vi "DiscArchiver.new event data.vi"(0 "i ref":refnum<vi>, 1 "eventData":string, 2 "descriptor":string, 3 "ms timeout (10000)":i32=10000, 5 "error in (no error)":errorcluster) -> (14 "i ref out":refnum<vi>, 17 "timed out":bool, 19 "error out":errorcluster)   [LabVIEW 2014, in "DiscArchiver.lvlib"]
doc: "The method is executed, when new event data is received. The data will be written to file."
uses:
  DiscArchiver.lvlib
  CS_Core/CSSystem/CoreDefs/CoreDefs.rawDataType.ctl
  CS_Core/CSSystem/CoreDefs/CoreDefs.error_type.ctl
  CS_Core/CSSystem/CoreDefs/CoreDefs.error_severity.ctl
  DataLib/DataLib.lvlib
  CS_Core/CSSystem/CoreLib/CoreLib.lvlib
  CSlibraries-extern/DimLVEvent/LVDimInterface/LVDimInterface.lvlib
  CSlibraries/UtilityLib/UtilityLib.lvlib
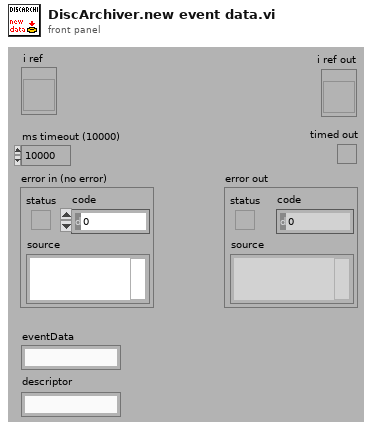
[diagram p1: front panel]
types:
  T1 = typedef "CoreDefs.rawDataType.ctl" = i8[]
  T2 = typedef "CoreDefs.error_severity.ctl" = enum16{"undefined", "information", "warning", "error", "fatal"}
  T3 = typedef "CoreDefs.error_type.ctl" = enum16{"no error", "can't load process", "can't unload process", "process does not exist", "can't install process", "can't remove process", "unknown function", "time out", "can't execute function", "duplicate queue name", "super not found", "caller queue invalid", "can't ping process", "unknown error", "VISA Error", "VISA timeout", "GPIB timeout", "GPIB error", "communication error", "data type mismatch", "can't read data from OPC server", "can't write data to OPC server", "OET error", "function not implemented", "process already exists", "invalid Shared Variable name", "error writing Shared Variable", "error reading Shared Variable", "invalid client name", "corrupt database", "unknown class", "call not authorized", "parameter out of range", "OET timeout: can't get data to modify", "invalid queue name", "requested operation incompatible with current state", "event undefined", "event disabled", "state undefined", "caller is not a friend", "EventBuilder: bad eventID", "EventBuilder: no DAQ devices", "a thread must not stop itself", "UNUSED ELEMENT4", "DiscArchiver: eventData incomplete", "DiscArchiver: eventData does not belong to run", "DiscArchiver: can't open file", "DiscArchiver: can't write to file", "DiscArchiver: available disc space low", "can't acquire semaphore", "error reading data from database", "notifier object is not existing", "can't register process", "can't unregister process", "illegal event type", "object disabled", "object already exists", "can't change state", "Instrument not found", "no connection to remote node", "invalid reference", "N/A", "UNUSED ELEMENT 1", "element not found", "illegal TCP/IP connection detected", "object does not exist", "invalid access ID", "unknown CS system", "invalid privilige", "unsupported data type", "unsupported server type", "IO server already exists", "Shared Variable already exists"}
  T4 = typedef "DiscArchiver.lvlib/DiscArchiver.i attribute.ctl" = cluster{"file prefix":string, "actual file":string, "nOfEvents":i32, "file":refnum<file>, "eventBuilder":string, "disc size alarm":bool, "dataDescription":string, "dataDescriptionURL":string, "eventDataURL":string, "headerID":dbl, "completeData":bool, "nOfEventsID":i32, "dataFileID":i32}
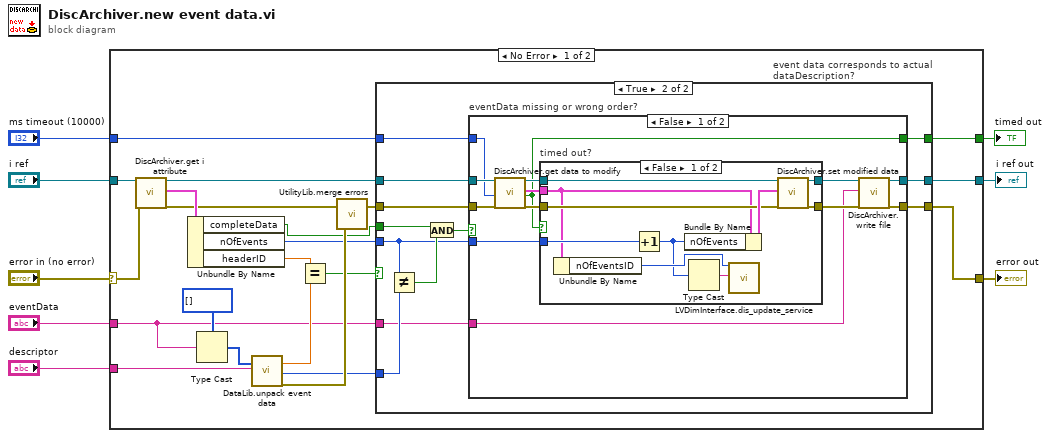
[diagram p0: block diagram]
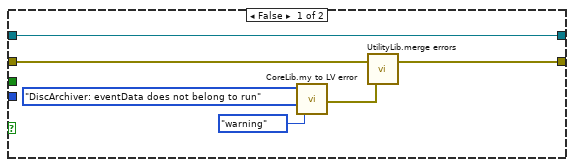
[diagram p2: hidden frame]
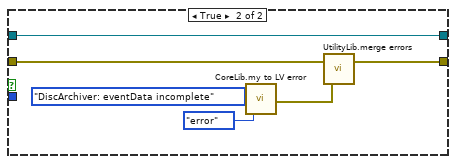
[diagram p4: hidden frame]
diagram:
  n1 = case shown="No Error" "error in (no error)" {
    selector: "error in (no error)" -> [w26 w79]
    tunnel: [w23 w79] -> w8
    tunnel: "eventData" -> [w9 _]
    tunnel: [w22 w80] -> w6
    tunnel: "i ref" -> [w27 w80]
    tunnel: "ms timeout (10000)" -> [w24 _]
    tunnel: "descriptor" -> [w17 _]
    tunnel: [w21 _] -> w2
    frame No Error {
      n2 = call "DiscArchiver.get i attribute.vi"("i ref in"=w27, "error in (no error)"=w26) -> ("i ref out"=w25:refnum<vi>, "i attribute"=w28:T4, "error out"=w15:errorcluster)  [unwired: 15 in]
      n3 = Unbundle By Name(w28) -> ("completeData"=w10:bool, "nOfEvents"=w12:i32, "headerID"=w29:dbl)
      n4 = Type Cast(type=T1 [] ("Array"), x=w9) -> (*(type *) &x=w20:T1)
      n5 = call "DataLib.unpack event data.vi"("serviceData"=w20, "descriptor"=w17) -> ("headerID"=w18:dbl, "eventID"=w11:i32, "error out"=w14:errorcluster)  [unwired: 13 in, 2 out]
      n6 = Equal?(x=w29, y=w18) -> (x = y?=w13:bool)
      n7 = call "UtilityLib.merge errors.vi"("error2 (no error)"=w14, "error1 (no error)"=w15) -> ("error out"=w16:errorcluster)
      n8 = case "event data corresponds to actual dataDescription?" shown="True" w13 {
        tunnel: w25 -> [w35 w47]
        tunnel: w16 -> [w32 w46]
        tunnel: w24 -> [_ w45]
        tunnel: [w33 w44] -> w23
        tunnel: [w35 w43] -> w22
        tunnel: [_ w42] -> w21
        tunnel: w12 -> [_ w37]
        tunnel: w11 -> [_ w41]
        tunnel: w10 -> [_ w40]
        tunnel: w9 -> [_ w36]
        frame False {
          n9 = call "CoreLib.my to LV error.vi"("ErrorTypes"=CoreDefs.error_type."DiscArchiver: eventData does not belong to run", "severityLevel"=CoreDefs.error_severity."warning") -> ("myErrorCluster"=w31:errorcluster)  [unwired: 16 in, 1 out]
          n10 = call "UtilityLib.merge errors.vi"("error2 (no error)"=w31, "error1 (no error)"=w32) -> ("error out"=w33:errorcluster)
        }
        frame True {
          n11 = Not Equal?(x=w37, y=w41) -> (x != y?=w39:bool)
          n12 = And(x=w40, y=w39) -> (x .and. y?=w38:bool)
          n13 = case "eventData missing or wrong order?" shown="False" w38 {
            tunnel: w47 -> [w60 w78]
            tunnel: w46 -> [w59 w76]
            tunnel: w45 -> [w53 _]
            tunnel: [w52 w77] -> w44
            tunnel: [w51 w78] -> w43
            tunnel: [w49 _] -> w42
            tunnel: w37 -> [w50 _]
            tunnel: w36 -> [w48 _]
            frame False {
              n14 = call "DiscArchiver.get data to modify.vi"("i ref in"=w60, "ms timeout (10000)"=w53, "error in (no error)"=w59) -> ("i ref out"=w58:refnum<vi>, "i attribute"=w57:T4, "timed out"=w49:bool, "error out"=w56:errorcluster)  [unwired: 13 in]
              n15 = case "timed out?" shown="False" w49 {
                tunnel: w58 -> [w70 w71]
                tunnel: w57 -> [w64 _]
                tunnel: w56 -> [w68 w72]
                tunnel: [w65 w72] -> w54
                tunnel: [w67 w71] -> w55
                tunnel: w50 -> [w66 _]
                frame False {
                  n16 = Unbundle By Name(w64) -> ("nOfEventsID"=w63:i32)
                  n17 = Increment(x=w66) -> (x+1=w61:i32)
                  n18 = Bundle By Name(cluster=w64, "nOfEvents"=w61) -> (w69:T4)
                  n19 = Type Cast(x=w61) -> (*(type *) &x=w62:string)  [unwired: 1 in]
                  n20 = call "LVDimInterface.dis_update_service.vi"("my_serviceID"=w63, "data"=w62) -> ()  [unwired: 15 in, 3 out]
                  n21 = call "DiscArchiver.set modified data.vi"("i ref in"=w70, "i attribute"=w69, "error in (no error)"=w68) -> ("i ref out"=w67:refnum<vi>, "error out"=w65:errorcluster)  [unwired: 15 in]
                }
                frame True {
                }
              }
              n22 = call "DiscArchiver.write file.vi"("i ref in"=w55, "eventData"=w48, "error in (no error)"=w54) -> ("i ref out"=w51:refnum<vi>, "error out"=w52:errorcluster)  [unwired: 15 in]
            }
            frame True {
              n23 = call "CoreLib.my to LV error.vi"("ErrorTypes"=CoreDefs.error_type."DiscArchiver: eventData incomplete", "severityLevel"=CoreDefs.error_severity."error") -> ("myErrorCluster"=w75:errorcluster)  [unwired: 16 in, 1 out]
              n24 = call "UtilityLib.merge errors.vi"("error2 (no error)"=w75, "error1 (no error)"=w76) -> ("error out"=w77:errorcluster)
            }
          }
        }
      }
    }
    frame Error {
    }
  }
  "error out" <- w8
  "i ref out" <- w6
  "timed out" <- w2
